vi "save.vi"(7 "description":string, 8 "error in (no error)":errorcluster, 9 "force format?":T1, 10 "path":path, 11 "Image in":refnum<class "Image.lvclass">) -> (0 "error out":errorcluster, 3 "Image out":refnum<class "Image.lvclass">)   [LabVIEW 2010, in "Image.lvclass"]
uses:
  Image.lvclass
  target_format_enum.ctl
  ErrorController/ErrorController/class_data.vi
  libraries/TIFFManagement/TIFFManagement.lvlib
  ErrorController/ErrorController/ErrorController.lvclass
panel:
  out "Intensity Graph":dbl[][](graph)
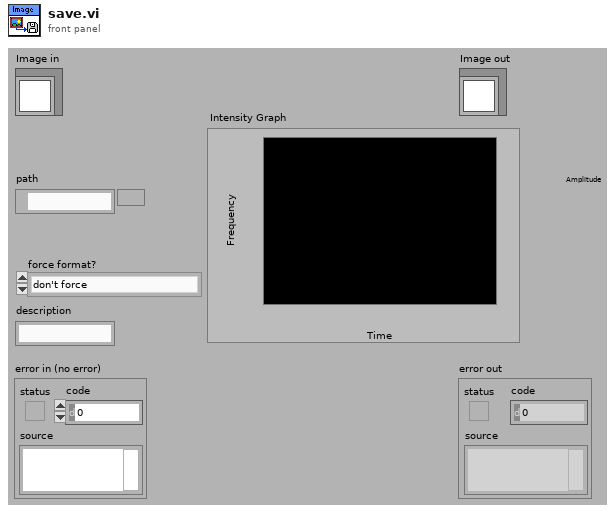
[diagram p1: front panel]
types:
  T1 = typedef "target_format_enum.ctl" = enum16{"don't force", "uint8", "uint16", "int16", "uint32", "int32", "single float"}
  T2 = typedef "Image Type" = u32
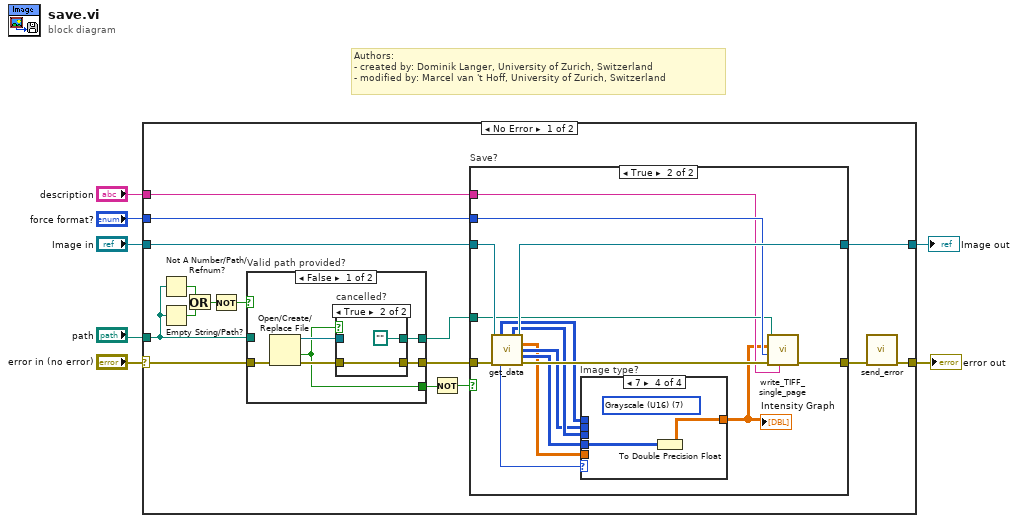
[diagram p0: block diagram]
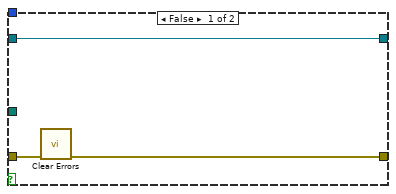
[diagram p2: hidden frame]
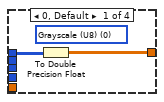
[diagram p3: hidden frame]
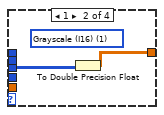
[diagram p4: hidden frame]
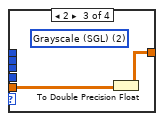
[diagram p5: hidden frame]
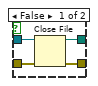
[diagram p6: hidden frame]
diagram:
  # "Authors: \n- created by: Dominik Langer, University of Zurich, Switzerland\n- modified by: Marcel van 't Hoff, University of Zurich, Switzerland"
  n1 = case shown="No Error" "error in (no error)" {
    selector: "error in (no error)" -> [w23 w65]
    tunnel: [w9 w65] -> w6
    tunnel: [w12 w64] -> w4
    tunnel: "Image in" -> [w14 w64]
    tunnel: "path" -> [w18 _]
    tunnel: "force format?" -> [w11 _]
    tunnel: "description" -> [w10 _]
    frame No Error {
      n2 = Not A Number/Path/Refnum?(number/path/refnum=w18) -> (NaN/Path/Refnum?=w21:bool)
      n3 = Empty String/Path?(string/path=w18) -> (empty?=w22:bool)
      n4 = Or(x=w21, y=w22) -> (x .or. y?=w20:bool)
      n5 = Not(x=w20) -> (.not. x?=w19:bool)
      n6 = case "Valid path provided?" shown="False" w19 {
        tunnel: w23 -> [w53 w63]
        tunnel: [w52 w63] -> w17
        tunnel: [w51 w62] -> w13
        tunnel: w18 -> [_ w62]
        tunnel: [w50 _] -> w16
        frame False {
          n7 = Open/Create/Replace File(error in=w53) -> (refnum out=w55:refnum<file>, cancelled=w50:bool, error out=w54:errorcluster)  [unwired: 5 in]
          n8 = case "cancelled?" shown="True" w50 {
            tunnel: w55 -> [w59 _]
            tunnel: w54 -> [w58 w60]
            tunnel: [w57 w60] -> w52
            tunnel: [w56 path ""] -> w51
            frame False {
              n9 = Close File(refnum=w59, error in=w58) -> (path=w56:path, error out=w57:errorcluster)
            }
            frame True {
            }
          }
        }
        frame True {
        }
      }
      n10 = Not(x=w16) -> (.not. x?=w15:bool)
      n11 = case "Save?" shown="True" w15 {
        tunnel: w17 -> [w25 w40]
        tunnel: [w24 w41] -> w8
        tunnel: w14 -> [w26 w38]
        tunnel: w13 -> [_ w29]
        tunnel: [w26 w37] -> w12
        tunnel: w11 -> [_ w30]
        tunnel: w10 -> [_ w28]
        frame False {
          n12 = call <vilib>:"Clear Errors.vi"("error in (no error)"=w25) -> ("error out"=w24:errorcluster)  [unwired: 6 in]
        }
        frame True {
          n13 = call-dynamic "get_data.vi"("Image in"=w38, "error in (no error)"=w40) -> ("Image Pixels (U8)"=w35:u8[][], "Image Pixels (I16)"=w34:i16[][], "Image out"=w37:refnum<class "Image.lvclass">, "Image Pixels (Float)"=w31:sgl[][], "Image Pixels (U16)"=w33:u16[][], "Image Pixels (U32)"=w32:u32[][], "Image Type"=w36:T2, "error out"=w39:errorcluster)  [unwired: 5 in, 1 out]
          n14 = case "Image type?" shown="7" w36 {
            tunnel: w35 -> [w43 _ _ _]
            tunnel: w34 -> [_ w44 _ _]
            tunnel: w33 -> [_ _ _ _]
            tunnel: w32 -> [_ _ _ w49]
            tunnel: w31 -> [_ _ w47 _]
            tunnel: [w42 w45 w46 w48] -> w27
            frame 0, Default {
              (unwired) T2 0 items=["Grayscale (U8)", "Grayscale (I16)", "Grayscale (SGL)", "Complex (CSG)", "RGB (U32)", "HSL (U32)", "RGB (U64)", "Grayscale (U16)"] ("Image Type")
              n15 = To Double Precision Float(number=w43) -> (double precision float=w42:dbl[][])
            }
            frame 1 {
              (unwired) T2 1 items=["Grayscale (U8)", "Grayscale (I16)", "Grayscale (SGL)", "Complex (CSG)", "RGB (U32)", "HSL (U32)", "RGB (U64)", "Grayscale (U16)"] ("Image Type")
              n16 = To Double Precision Float(number=w44) -> (double precision float=w45:dbl[][])
            }
            frame 2 {
              (unwired) T2 2 items=["Grayscale (U8)", "Grayscale (I16)", "Grayscale (SGL)", "Complex (CSG)", "RGB (U32)", "HSL (U32)", "RGB (U64)", "Grayscale (U16)"] ("Image Type")
              n17 = To Double Precision Float(number=w47) -> (double precision float=w46:dbl[][])
            }
            frame 7 {
              (unwired) T2 7 items=["Grayscale (U8)", "Grayscale (I16)", "Grayscale (SGL)", "Complex (CSG)", "RGB (U32)", "HSL (U32)", "RGB (U64)", "Grayscale (U16)"] ("Image Type")
              n18 = To Double Precision Float(number=w49) -> (double precision float=w48:dbl[][])
            }
          }
          "Intensity Graph" <- w27
          n19 = call "write_TIFF_single_page.vi"("description"=w28, "error in (no error)"=w39, "force format?"=w30, "data"=w27, "path in"=w29) -> ("error out"=w41:errorcluster)  [unwired: 5 in, 1 out]
        }
      }
      n20 = call "send_error.vi"("error in (no error)"=w8) -> ("error out"=w9:errorcluster)  [unwired: 10 in]
    }
    frame Error {
    }
  }
  "error out" <- w6
  "Image out" <- w4
